vi "State Machine Automation.vi"() -> ()   [LabVIEW 2016]
panel:
  in  "Path":path=path "C:/Users/monke/OneDrive/Documents/Research/Repository/automation/itx folders/Destination Files"
  in  "Tab Control":enum32{"Conductance", "Transconductance"}(tab)
  out "Conductance":T1(graph)
  out "Cond. Intens. 2":dbl[][](graph)
  out "Transconductance":T1(graph)
  out "Trans. Intens. 2":dbl[][](graph)
  in  "STOP":bool
  out "Added?":string
  in  "Numeric":dbl=20.0
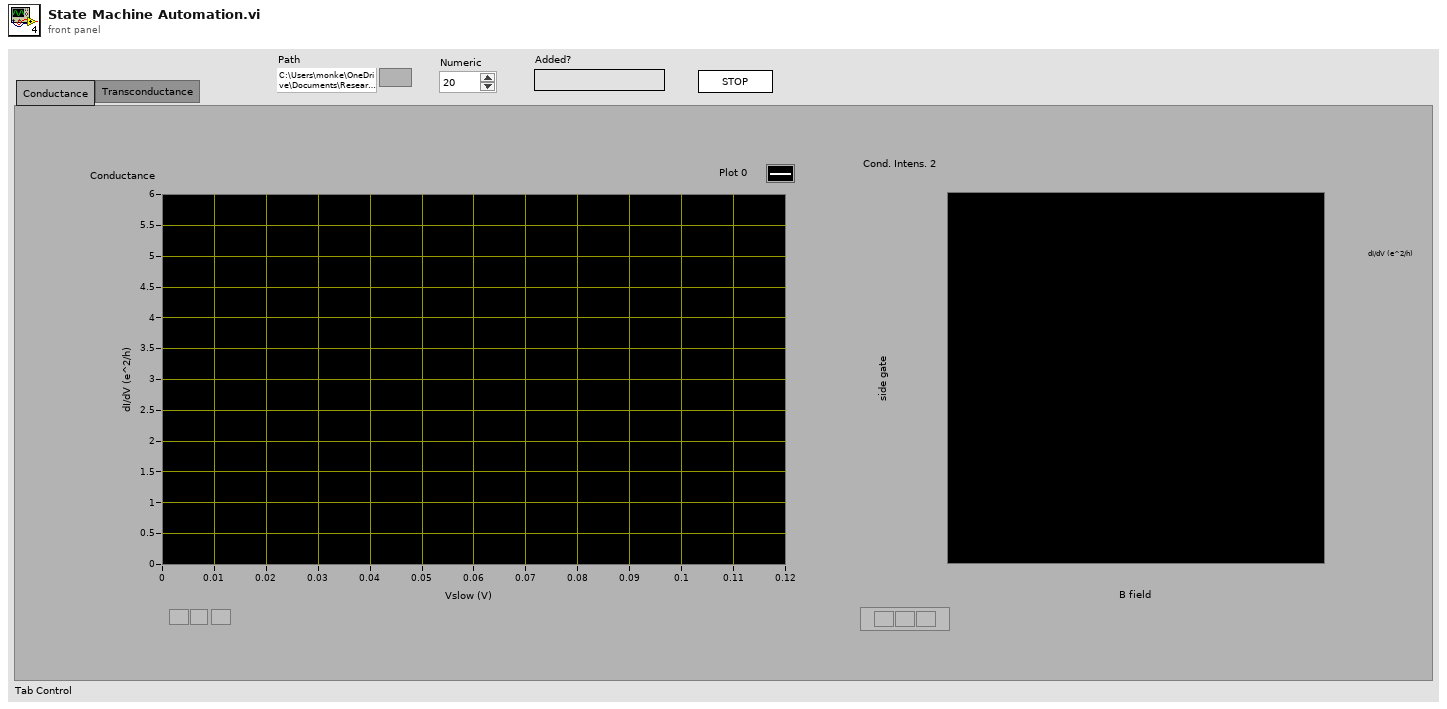
[diagram p1: front panel]
types:
  T1 = cluster{"Vfast":dbl[], "Decimated Array":dbl[]}[]
  T2 = enum32{"invalid app kind", "Development System", "Run Time System", "Student Edition", "Embedded LabVIEW", "Evaluation", "Custom"}
  T3 = enum32{"Invalid", "Standard", "Closed", "Hidden", "Minimized", "Maximized"}
  T4 = cluster{"Core":cluster{"Current VI Reference":refnum<vi>, "Close Panel on Exit?":bool}, "Your Boolean data":bool, "Your string data":string, "Path":path, "Normal Graphs":cluster{"A vs D":cluster{dbl[], dbl[]}[], "Transconductance 2":cluster{"Vfast":dbl[], "Decimated Array":dbl[]}[], "Start Up":cluster{dbl[], dbl[]}[]}, "Intensity Graphs":cluster{"Cond. Intens. 3":dbl[][], "Trans. Intens. 3":dbl[][]}, "offset":i32}
  T5 = cluster{"Cond. Intens. 3":dbl[][], "Trans. Intens. 3":dbl[][]}
  T6 = cluster{"A vs D":cluster{dbl[], dbl[]}[], "Transconductance 2":cluster{"Vfast":dbl[], "Decimated Array":dbl[]}[], "Start Up":cluster{dbl[], dbl[]}[]}
  T7 = cluster{"Current VI Reference":refnum<vi>, "Close Panel on Exit?":bool}
  T8 = cluster{"Decimated Array":dbl[], "Decimated Array":dbl[]}
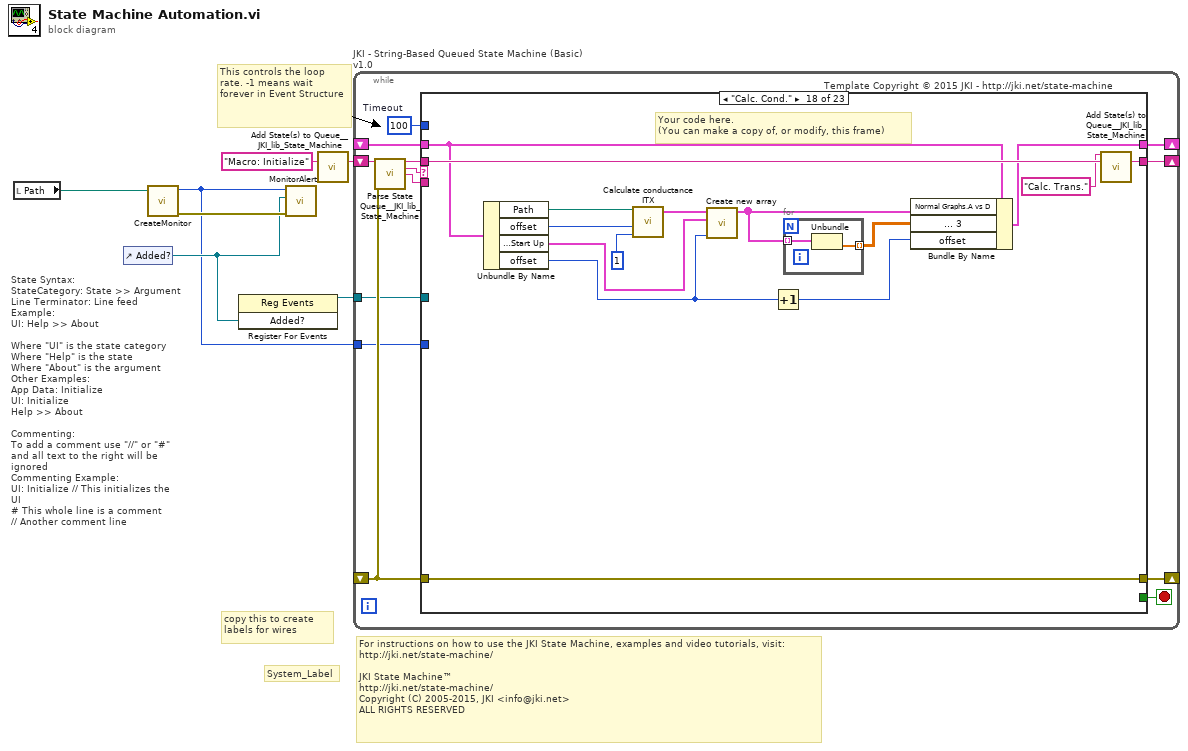
[diagram p0: block diagram]
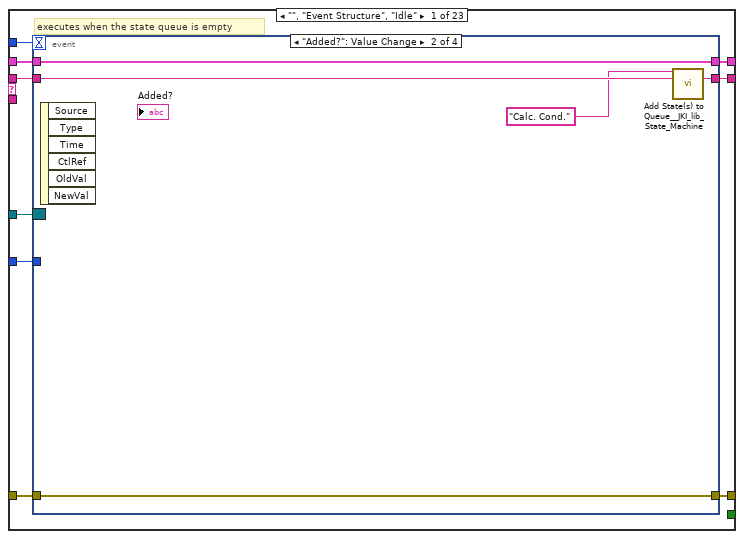
[diagram p2: hidden frame]
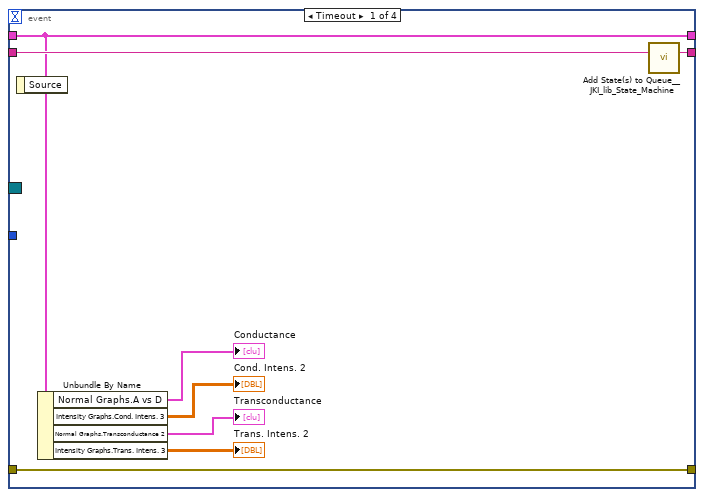
[diagram p3: hidden frame]
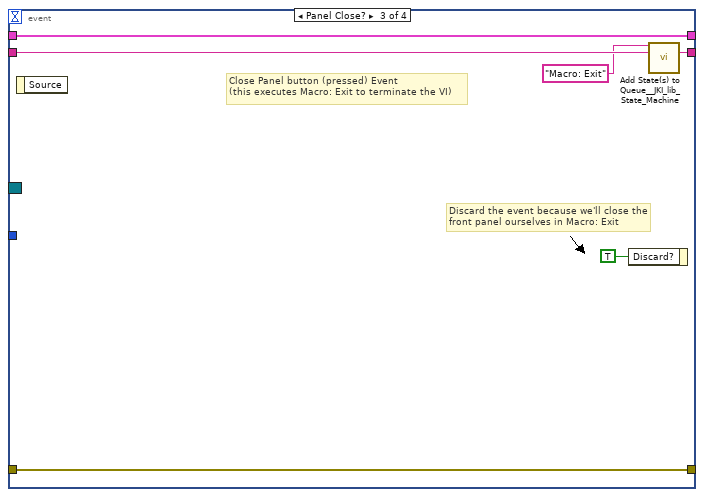
[diagram p4: hidden frame]
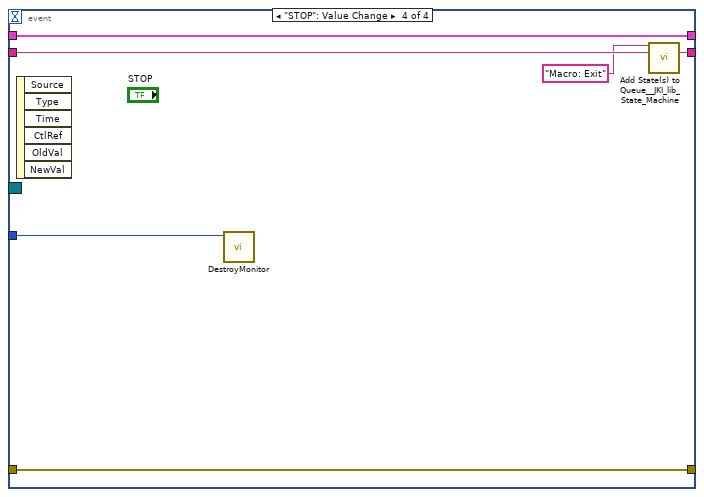
[diagram p5: hidden frame]
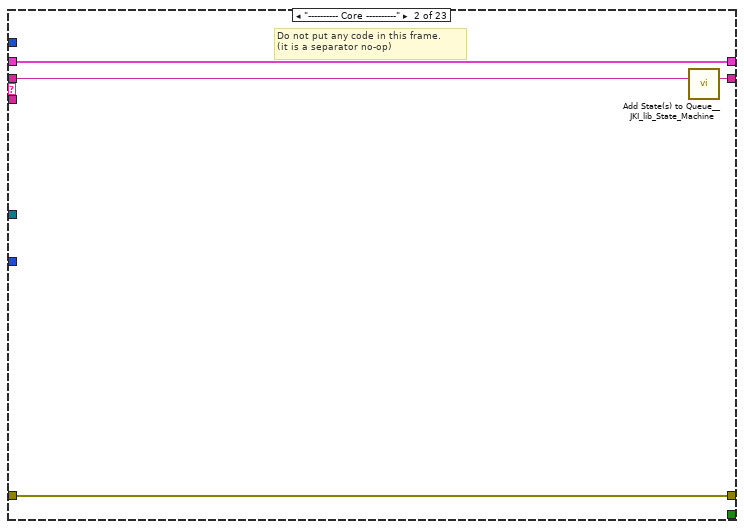
[diagram p6: hidden frame]
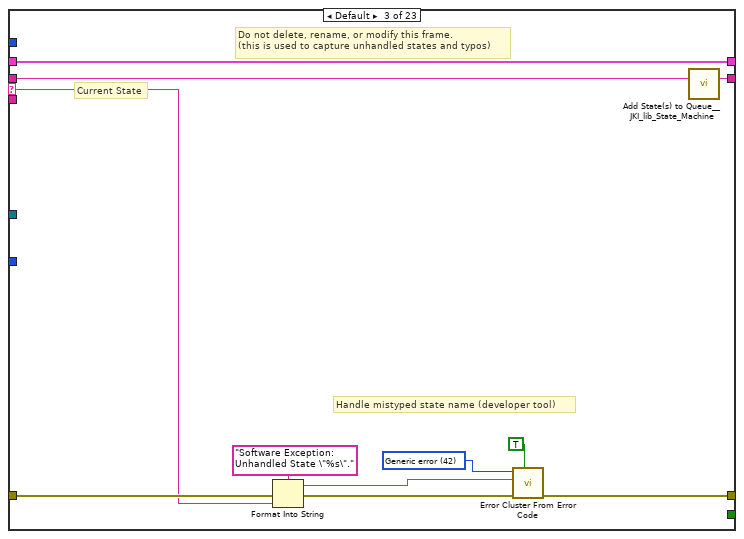
[diagram p7: hidden frame]
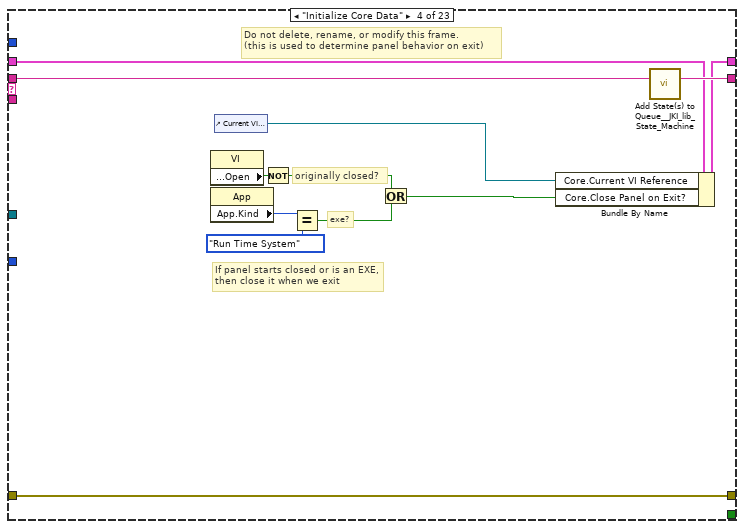
[diagram p8: hidden frame]
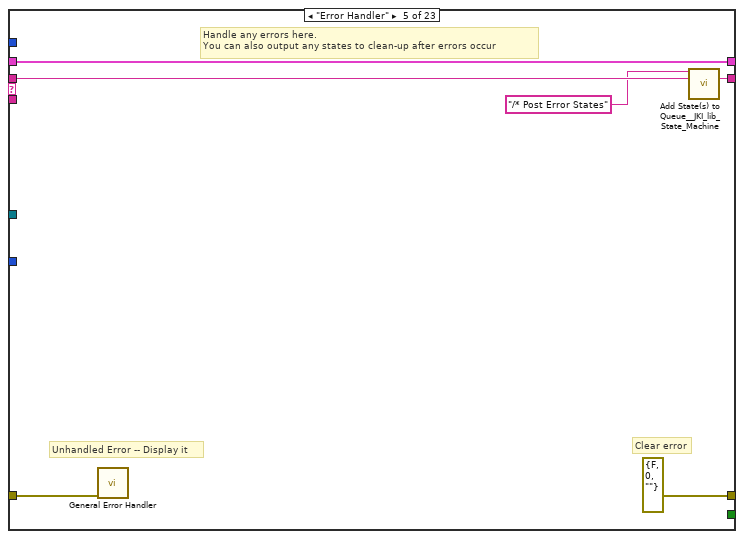
[diagram p9: hidden frame]
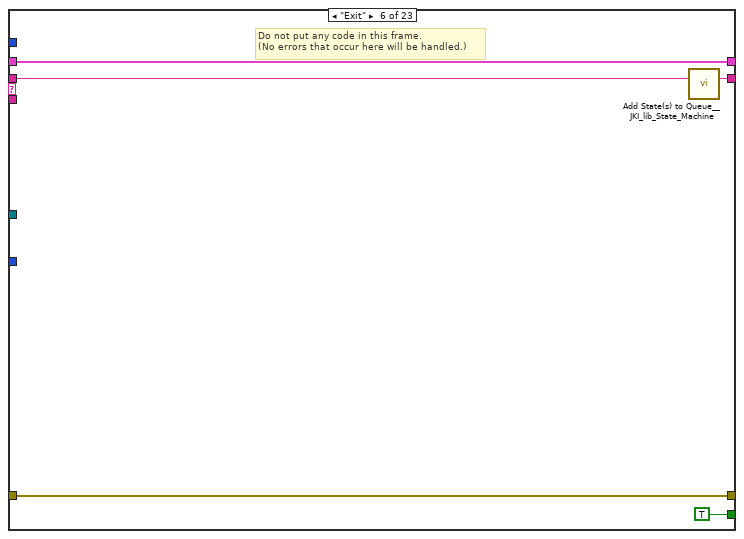
[diagram p10: hidden frame]
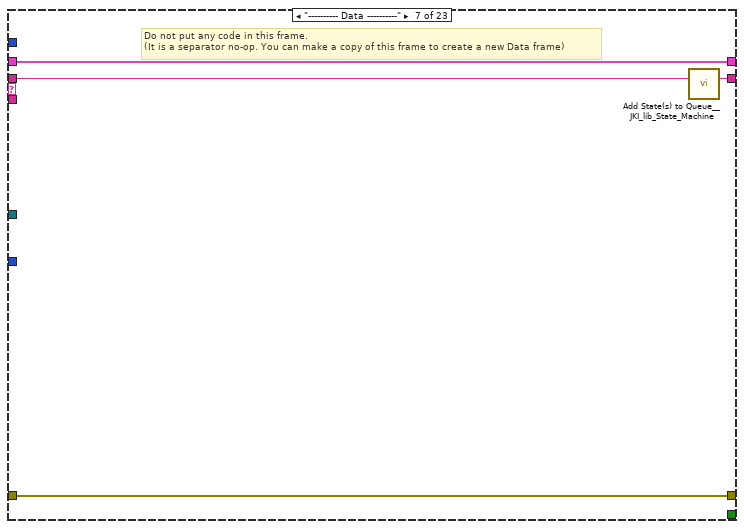
[diagram p11: hidden frame]
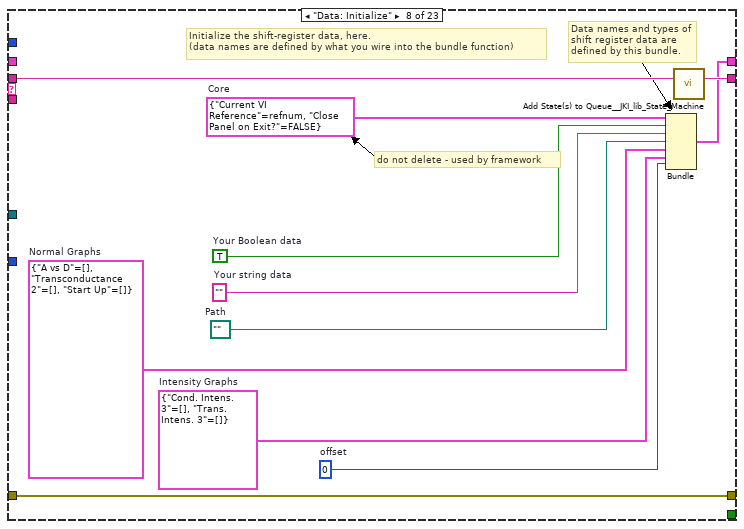
[diagram p12: hidden frame]
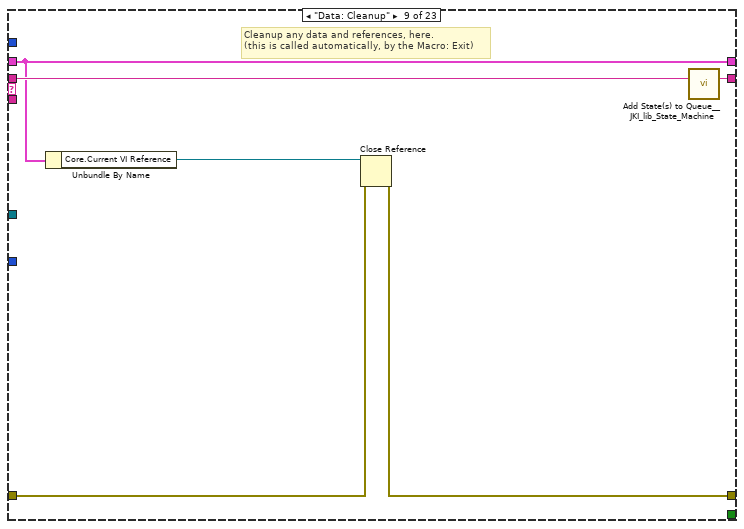
[diagram p13: hidden frame]
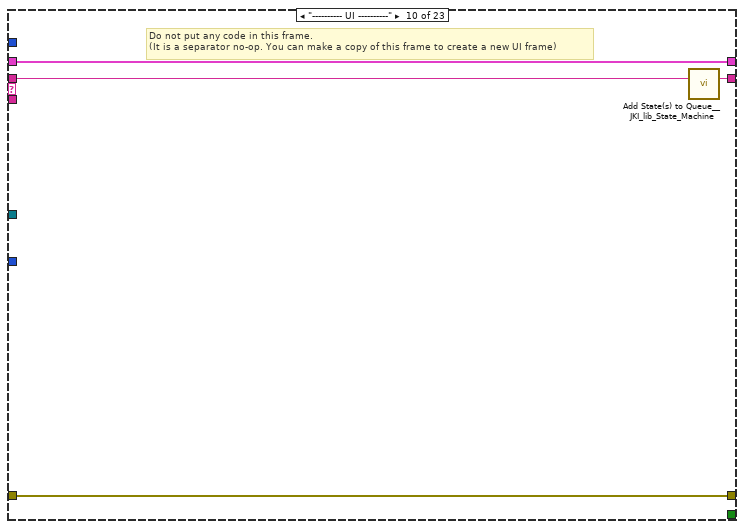
[diagram p14: hidden frame]
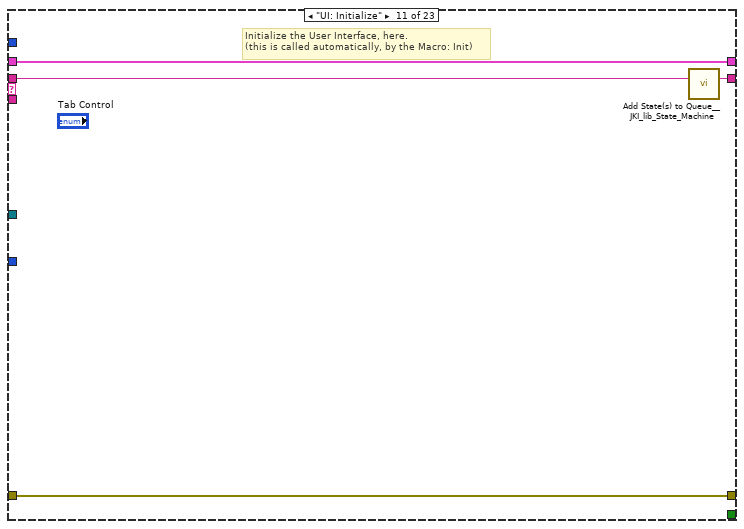
[diagram p15: hidden frame]
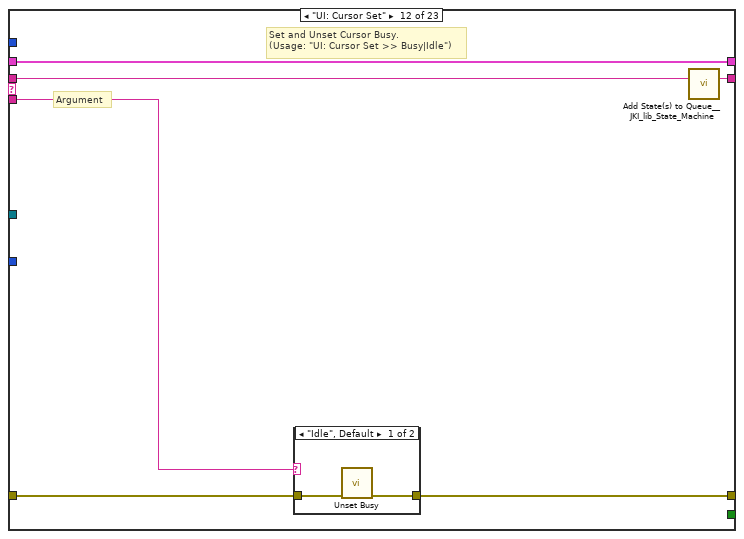
[diagram p16: hidden frame]
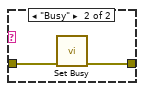
[diagram p17: hidden frame]
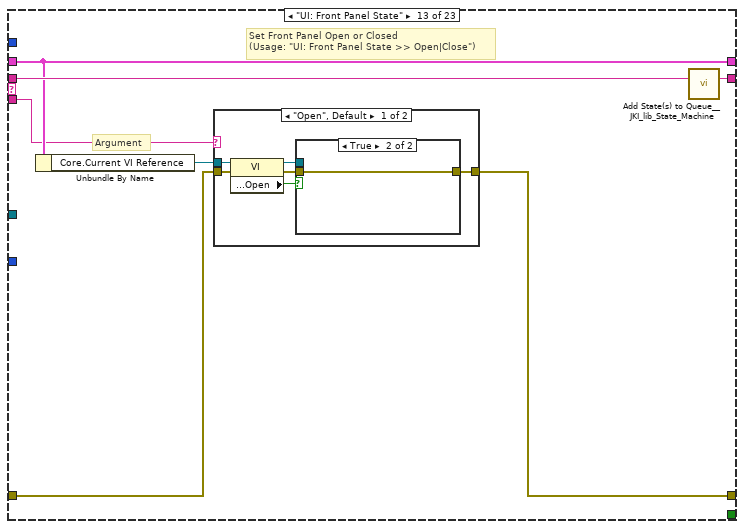
[diagram p18: hidden frame]
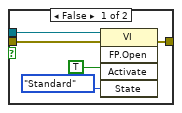
[diagram p19: hidden frame]
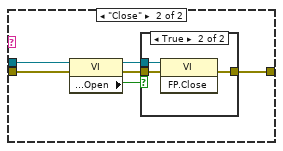
[diagram p20: hidden frame]
diagram:
  # "For instructions on how to use the JKI State Machine, examples and video tutorials, visit:\nhttp://jki.net/state-machine/\n\nJKI State Machine™\nhttp://jki.net/state-machine/\nCopyright (C) 2005-2015, JKI <info@jki.net>\nALL RIGHTS RESERVED"
  # "State Syntax:\nStateCategory: State >> Argument\nLine Terminator: Line feed\nExample:\nUI: Help >> About\n\nWhere \"UI\" is the state category\nWhere \"Help\" is the state\nWhere \"About\" is the argument\nOther Examples:\nApp Data: Initialize\nUI: Initialize\nHelp >> About\n\nCommenting:\nTo add a comment use \"//\" or \"#\" and all text to the right will be ignored\nCommenting Example:\nUI: Initialize // This initializes the UI\n# This whole line is a comment\n// Another comment line"
  # "copy this to create labels for wires"
  # "This controls the loop rate. -1 means wait forever in Event Structure"
  # "System_Label"
  n1 = local read "Path"() -> (w1:path)
  n2 = control-ref of="Added?"() -> (w4:refnum<vi>)
  n3 = call "CreateMonitor.vi"("File Path Control"=w1) -> ("error out"=w5:errorcluster, "Handle"=w2:i32)  [unwired: 9 in]
  n4 = register-events(w4) -> (reference out=w3:refnum<event-registration>)  [unwired: 2 in, 1 out]
  n5 = call "MonitorAlert.vi"("error in (no error)"=w5, "Str Refnum"=w4, "Handle"=w2) -> ()  [unwired: 8 in, 1 out]
  n6 = call <vilib>:"Add State(s) to Queue__JKI_lib_State_Machine.vi"("State(s) in (\"\")"="Macro: Initialize") -> ("States Out"=w7:string)  [unwired: 14 in]
  n7 = while "JKI - String-Based Queued State Machine (Basic) v1.0" {
    shift-right: [w13] -> _
    shift-left: _ -> [w12]
    shift-right: [w16] -> _
    shift-left: _ -> [w10]
    shift-right: [w15] -> _
    shift-left: w7 -> [w17]
    tunnel: w3 -> [w9]
    tunnel: w2 -> [w8]
    stop <- w14 stop-if-true
    w11 = 100  # Timeout
    # "Template Copyright © 2015 JKI - http://jki.net/state-machine"
    n8 = call <vilib>:"Parse State Queue__JKI_lib_State_Machine.vi"("State Queue"=w17, "Error In (no error)"=w10) -> ("Remaining States"=w19:string, "Current State"=w20:string, "Arguments"=w18:string)  [unwired: 11 in]
    n9 = case shown="\"Calc. Cond.\"" w20 {
      selector: w20 -> [_ _ w59 _ _ _ _ _ _ _ _ _ _ _ _ _ _ _ _ _ _ _ _]
      tunnel: w19 -> [w29 w58 w63 w81 w87 w92 w96 w107 w113 w117 w121 w127 w138 w164 w169 w179 w183 w198 w208 w217 w227 w231 w235]
      tunnel: w18 -> [_ _ _ _ _ _ _ _ _ _ _ w122 w132 _ _ _ _ _ _ _ _ _ _]
      tunnel: w12 -> [w27 w55 w61 w72 w84 w90 w93 _ w108 w114 w119 w125 w134 w161 w166 w176 w180 w194 w202 w214 w219 w228 w232]
      tunnel: [w26 w56 w65 w78 errorcluster {"status"=FALSE, "code"=0, "source"=""} ("error out") w89 w94 w104 w109 w115 w118 w123 w135 w162 w167 w177 w181 w196 w206 w215 w225 w229 w233] -> w16
      tunnel: w10 -> [w25 w56 w64 w78 w83 w89 w94 w104 w110 w115 w118 w124 w136 w162 w167 w177 w181 w196 w206 w215 w225 w229 w233]
      tunnel: [w28 w57 w62 w80 w86 w91 w95 w106 w112 w116 w120 w126 w137 w163 w168 w178 w182 w197 w207 w216 w226 w230 w234] -> w15
      tunnel: [_ _ _ _ _ TRUE _ _ _ _ _ _ _ _ _ _ _ _ _ _ _ _ _] -> w14
      tunnel: [w24 w55 w61 w79 w84 w90 w93 w105 w108 w114 w119 w125 w134 w161 w166 w176 w180 w193 w201 w214 w224 w228 w232] -> w13
      tunnel: w11 -> [w23 _ _ _ _ _ _ _ _ _ _ _ _ _ _ _ _ _ _ _ _ _ _]
      tunnel: w9 -> [w22 _ _ _ _ _ _ _ _ _ _ _ _ _ _ _ _ _ _ _ _ _ _]
      tunnel: w8 -> [w21 _ _ _ _ _ _ _ _ _ _ _ _ _ _ _ _ _ _ _ _ _ _]
      frame "", "Event Structure", "Idle" {
        # "executes when the state queue is empty"
        n10 = event shown="[1] \"Added?\": Value Change" {
          selector: w22 -> [_ _ _ _]
          dyn-events: _ -> [_ _ _ _]
          timeout: w23 -> [_ _ _ _]
          tunnel: w29 -> [w37 w42 w48 w54]
          tunnel: [w36 w41 w47 w53] -> w28
          tunnel: w27 -> [w30 w39 w45 w51]
          tunnel: [w35 w40 w46 w52] -> w26
          tunnel: w25 -> [w35 w40 w46 w52]
          tunnel: [w30 w39 w45 w51] -> w24
          tunnel: w21 -> [_ _ _ w49]
          event Timeout {
            n11 = event-data() -> ()  [unwired: 1 in, 1 out]
            n12 = Unbundle By Name(w30) -> ("Normal Graphs.A vs D"=→"Conductance":cluster{dbl[], dbl[]}[], "Intensity Graphs.Cond. Intens. 3"=→"Cond. Intens. 2":dbl[][], "Normal Graphs.Transconductance 2"=→"Transconductance":T1, "Intensity Graphs.Trans. Intens. 3"=→"Trans. Intens. 2":dbl[][])
            n13 = call <vilib>:"Add State(s) to Queue__JKI_lib_State_Machine.vi"("State(s) in (\"\")"=w37) -> ("States Out"=w36:string)  [unwired: 14 in]
          }
          event "Added?": Value Change {
            n14 = event-data() -> ()  [unwired: 1 in, 6 out]
            n15 = call <vilib>:"Add State(s) to Queue__JKI_lib_State_Machine.vi"("State(s) in Front (\"\")"="Calc. Cond." ("State(s) in Front (\"\")"), "State(s) in (\"\")"=w42) -> ("States Out"=w41:string)  [unwired: 13 in]
          }
          event Panel Close? {
            # "Discard the event because we'll close the front panel ourselves in Macro: Exit"
            # "Close Panel button (pressed) Event\n(this executes Macro: Exit to terminate the VI)"
            n16 = event-data() -> ()  [unwired: 1 in, 1 out]
            n17 = event-data("Discard?"=TRUE) -> ()  [unwired: 1 in, 1 out]
            n18 = call <vilib>:"Add State(s) to Queue__JKI_lib_State_Machine.vi"("State(s) in Front (\"\")"="Macro: Exit", "State(s) in (\"\")"=w48) -> ("States Out"=w47:string)  [unwired: 13 in]
          }
          event "STOP": Value Change {
            n19 = event-data() -> ()  [unwired: 1 in, 6 out]
            n20 = call "DestroyMonitor.vi"("Handle in"=w49) -> ()  [unwired: 10 in, 1 out]
            n21 = call <vilib>:"Add State(s) to Queue__JKI_lib_State_Machine.vi"("State(s) in Front (\"\")"="Macro: Exit", "State(s) in (\"\")"=w54) -> ("States Out"=w53:string)  [unwired: 13 in]
          }
        }
      }
      frame "---------- Core ----------" {
        # "Do not put any code in this frame.\n(it is a separator no-op)"
        n22 = call <vilib>:"Add State(s) to Queue__JKI_lib_State_Machine.vi"("State(s) in (\"\")"=w58) -> ("States Out"=w57:string)  [unwired: 14 in]
      }
      frame Default {
        w68 = 42 items=["No error", "Argument error", "Memory is full", "Out of zone", "End of file", "File already open", "Generic file I/O error", "File not found", "File permission error", "Disk is full", "Duplicate path", "Too many files open", "System feature not enabled", "Resource file not found", "Cannot add resource", "Resource not found", "Image not found", "Image memory error", "Pen does not exist", "Config type invalid", "Config token not found", "Config parse error", "Config memory error", "Bad external code format", "Bad external code offset", "External code not present", "Null window", "Destroy window error", "Null menu", "Print aborted", "Bad print record", "Print driver error", "Windows error during printing", "Memory error during printing", "Print dialog error", "Generic print error", "Invalid device refnum", "Device not found", "Device parameter error", "Device unit error", "Cannot open device", "Device call aborted", "Generic error", "Cancelled by user", "Object ID too low", "Object ID too high", "Object not in heap", "Unknown heap", "Unknown object (invalid DefProc)", "Unknown object (DefProc not in table)", "Message out of range", "Invalid (null) method", "Unknown message", "Manager call not supported", "Bad address", "Network operation in progress", "Network operation timed out", "Connection is busy", "Network attribute not supported", "Network error", "Address in use", "System out of memory", "Connection aborted", "Connection refused", "Not connected", "Already connected", "Connection closed", "Initialization error (interapplication manager)", "Bad occurrence", "Wait on unbound occurrence handler", "Occurrence queue overflow", "Datalog type conflict", "Unused", "Unrecognized type (interapplication manager)", "Memory corrupt", "Failed to make temporary DLL", "Old CIN version", "Drag socket not found", "Failed to load drop-object", "Failed to register OLE object", "Failed to release OLE object", "Format specifier type mismatch", "Unknown format specifier", "Too few format specifiers", "Too many format specifiers", "Scan failed", "Newer CIN version", "Error converting to variant", "Runtime menu error", "Password tampered", "Variant attribute not found", "Incompatible variant data type", "Event data is not available", "Event Store is not present", "Occurrence is not found", "Event Queue is not created", "Event info is not available", "Refnum passed is NULL", "Error retrieving Class GUID", "Error retrieving CoClass GUID", "Error retrieving TypeLib GUID.", "Bad built application magic bytes.", "Specific driver is different from the specific driver associated with the Logical Name.", "There is no session opened to the class driver.", "Max Error", "MAX - Error with config objects", "MAX - Error loading configuration", "MAX - Group not supported"]
        # "Current State"
        # "Do not delete, rename, or modify this frame.\n(this is used to capture unhandled states and typos)"
        # "Handle mistyped state name (developer tool)"
        n23 = Format Into String(format string="Software Exception: Unhandled State \"%s\"." ("message"), error in=w64, w59) -> (resulting string=w67:string, error out=w66:errorcluster)  [unwired: 1 in]
        n24 = call <vilib>:"Error Cluster From Error Code.vi"("show call chain? (False)"=TRUE, "error in (no error)"=w66, "error message (\"\")"=w67, "error code (0)"=w68) -> ("error out"=w65:errorcluster)  [unwired: 5 in]
        n25 = call <vilib>:"Add State(s) to Queue__JKI_lib_State_Machine.vi"("State(s) in (\"\")"=w63) -> ("States Out"=w62:string)  [unwired: 14 in]
      }
      frame "Initialize Core Data" {
        # "Do not delete, rename, or modify this frame.\n(this is used to determine panel behavior on exit)"
        # "originally closed?"
        # "exe?"
        # "If panel starts closed or is an EXE, then close it when we exit"
        n26 = property class="VI"() -> ("Front Panel.Open"=w77:bool)  [unwired: 2 in, 2 out]
        n27 = property class="App"() -> ("App.Kind"=w76:T2)  [unwired: 2 in, 2 out]
        n28 = control-ref of="Current VI Reference"() -> (w70:refnum<vi>)
        n29 = Not(x=w77) -> (.not. x?=w74:bool)
        n30 = Equal?(x=w76, y=T2."Run Time System" ("Application:Kind")) -> (x = y?=w73:bool)
        n31 = Or(x=w74, y=w73) -> (x .or. y?=w71:bool)
        n32 = Bundle By Name(cluster=w72, "Core.Current VI Reference"=w70, "Core.Close Panel on Exit?"=w71) -> (w79:T4)
        n33 = call <vilib>:"Add State(s) to Queue__JKI_lib_State_Machine.vi"("State(s) in (\"\")"=w81) -> ("States Out"=w80:string)  [unwired: 14 in]
      }
      frame "Error Handler" {
        # "Unhandled Error -- Display it"
        # "Handle any errors here.\nYou can also output any states to clean-up after errors occur"
        # "Clear error"
        n34 = call <vilib>:"General Error Handler.vi"("error in (no error)"=w83) -> ()  [unwired: 10 in, 5 out]
        n35 = call <vilib>:"Add State(s) to Queue__JKI_lib_State_Machine.vi"("State(s) in Front (\"\")"="/* Post Error States", "State(s) in (\"\")"=w87) -> ("States Out"=w86:string)  [unwired: 13 in]
      }
      frame "Exit" {
        # "Do not put any code in this frame.\n(No errors that occur here will be handled.)"
        n36 = call <vilib>:"Add State(s) to Queue__JKI_lib_State_Machine.vi"("State(s) in (\"\")"=w92) -> ("States Out"=w91:string)  [unwired: 14 in]
      }
      frame "---------- Data ----------" {
        # "Do not put any code in this frame.\n(It is a separator no-op. You can make a copy of this frame to create a new Data frame)"
        n37 = call <vilib>:"Add State(s) to Queue__JKI_lib_State_Machine.vi"("State(s) in (\"\")"=w96) -> ("States Out"=w95:string)  [unwired: 14 in]
      }
      frame "Data: Initialize" {
        w97 = 0  # offset
        w98 = T5 {"Cond. Intens. 3"=[], "Trans. Intens. 3"=[]}  # Intensity Graphs
        w99 = T6 {"A vs D"=[], "Transconductance 2"=[], "Start Up"=[]}  # Normal Graphs
        w100 = path ""  # Path
        w101 = T7 {"Current VI Reference"=refnum, "Close Panel on Exit?"=FALSE}  # Core
        w103 = TRUE  # Your Boolean data
        w102 = ""  # Your string data
        # "do not delete - used by framework"
        # "Data names and types of shift register data are defined by this bundle."
        # "Initialize the shift-register data, here.\n(data names are defined by what you wire into the bundle function)"
        n38 = Bundle("Core"=w101, "Your Boolean data"=w103, "Your string data"=w102, "Path"=w100, "Normal Graphs"=w99, "Intensity Graphs"=w98, "offset"=w97) -> (w105:T4)  [unwired: 1 in]
        n39 = call <vilib>:"Add State(s) to Queue__JKI_lib_State_Machine.vi"("State(s) in (\"\")"=w107) -> ("States Out"=w106:string)  [unwired: 14 in]
      }
      frame "Data: Cleanup" {
        # "Cleanup any data and references, here.\n(this is called automatically, by the Macro: Exit)"
        n40 = Unbundle By Name(w108) -> ("Core.Current VI Reference"=w111:refnum<vi>)
        n41 = Close Reference(reference=w111, error in (no error)=w110) -> (error out=w109:errorcluster)
        n42 = call <vilib>:"Add State(s) to Queue__JKI_lib_State_Machine.vi"("State(s) in (\"\")"=w113) -> ("States Out"=w112:string)  [unwired: 14 in]
      }
      frame "---------- UI ----------" {
        # "Do not put any code in this frame.\n(It is a separator no-op. You can make a copy of this frame to create a new UI frame)"
        n43 = call <vilib>:"Add State(s) to Queue__JKI_lib_State_Machine.vi"("State(s) in (\"\")"=w117) -> ("States Out"=w116:string)  [unwired: 14 in]
      }
      frame "UI: Initialize" {
        # "Initialize the User Interface, here.\n(this is called automatically, by the Macro: Init)"
        n44 = call <vilib>:"Add State(s) to Queue__JKI_lib_State_Machine.vi"("State(s) in (\"\")"=w121) -> ("States Out"=w120:string)  [unwired: 14 in]
      }
      frame "UI: Cursor Set" {
        # "Argument"
        # "Set and Unset Cursor Busy.\n(Usage: \"UI: Cursor Set >> Busy|Idle\")"
        n45 = case shown="\"Idle\", Default" w122 {
          tunnel: w124 -> [w129 w131]
          tunnel: [w128 w130] -> w123
          frame "Idle", Default {
            n46 = call <vilib>:"Unset Busy.vi"("error in (no error)"=w129) -> ("error out"=w128:errorcluster)  [unwired: 10 in]
          }
          frame "Busy" {
            n47 = call <vilib>:"Set Busy.vi"("error in (no error)"=w131) -> ("error out"=w130:errorcluster)  [unwired: 9 in, 1 out]
          }
        }
        n48 = call <vilib>:"Add State(s) to Queue__JKI_lib_State_Machine.vi"("State(s) in (\"\")"=w127) -> ("States Out"=w126:string)  [unwired: 14 in]
      }
      frame "UI: Front Panel State" {
        # "Argument"
        # "Set Front Panel Open or Closed\n(Usage: \"UI: Front Panel State >> Open|Close\")"
        n49 = Unbundle By Name(w134) -> ("Core.Current VI Reference"=w133:refnum<vi>)
        n50 = case shown="\"Open\", Default" w132 {
          tunnel: w136 -> [w142 w155]
          tunnel: [w144 w156] -> w135
          tunnel: w133 -> [w143 w153]
          frame "Open", Default {
            n51 = property class="VI"(reference=w143, error in=w142) -> (reference out=w140:refnum<vi>, error out=w141:errorcluster, "Front Panel.Open"=w139:bool)
            n52 = case shown="True" w139 {
              tunnel: [w147 w150] -> w144
              tunnel: w141 -> [w146 w150]
              tunnel: w140 -> [w145 _]
              frame False {
                n53 = invoke class="VI" method="FP.Open"(reference=w145, error in=w146, "Activate"=TRUE, "State"=T3."Standard") -> (error out=w147:errorcluster)  [unwired: 1 in, 4 out]
              }
              frame True {
              }
            }
          }
          frame "Close" {
            n54 = property class="VI"(reference=w153, error in=w155) -> (reference out=w152:refnum<vi>, error out=w154:errorcluster, "Front Panel.Open"=w151:bool)
            n55 = case shown="True" w151 {
              tunnel: [w157 w160] -> w156
              tunnel: w154 -> [w157 w159]
              tunnel: w152 -> [_ w158]
              frame False {
              }
              frame True {
                n56 = invoke class="VI" method="FP.Close"(reference=w158, error in=w159) -> (error out=w160:errorcluster)  [unwired: 1 in, 2 out]
              }
            }
          }
        }
        n57 = call <vilib>:"Add State(s) to Queue__JKI_lib_State_Machine.vi"("State(s) in (\"\")"=w138) -> ("States Out"=w137:string)  [unwired: 14 in]
      }
      frame "---------- Macro ----------" {
        # "Do not put any code in this frame.\n(It is a separator no-op. You can make a copy of this frame to create a new Macro frame)"
        n58 = call <vilib>:"Add State(s) to Queue__JKI_lib_State_Machine.vi"("State(s) in (\"\")"=w164) -> ("States Out"=w163:string)  [unwired: 14 in]
      }
      frame "Macro: Initialize" {
        # "Initialization Macro\n(This is called once, when the VI starts)"
        n59 = call <vilib>:"Add State(s) to Queue__JKI_lib_State_Machine.vi"("State(s) in Front (\"\")"="Data: Initialize\nInitialize Core Data\nUI: Initialize\nUI: Front Panel State >> Open\nCond.StartUp", "State(s) in (\"\")"=w169) -> ("States Out"=w168:string)  [unwired: 13 in]
      }
      frame "Macro: Exit" {
        # "Exit Macro\n(This is called once, when the VI exits)"
        n60 = Unbundle By Name(w176) -> ("Core.Close Panel on Exit?"=w175:bool)
        n61 = Select(t="UI: Front Panel State >> Close", s=w175, f="") -> (s? t:f=w172:string)
        n62 = call <vilib>:"Add State(s) to Queue__JKI_lib_State_Machine.vi"("State(s) in (\"\")"=w172, "State(s) at Back (\"\")"="Data: Cleanup\nExit") -> ("States Out"=w170:string)  [unwired: 13 in]
        n63 = call <vilib>:"Add State(s) to Queue__JKI_lib_State_Machine.vi"("State(s) in Front (\"\")"=w170, "State(s) in (\"\")"=w179) -> ("States Out"=w178:string)  [unwired: 13 in]
      }
      frame "---------- Cond. Trans. ----------" {
        # "Template Separator\n(You can make a copy of, or modify, this frame)"
        n64 = call <vilib>:"Add State(s) to Queue__JKI_lib_State_Machine.vi"("State(s) in (\"\")"=w183) -> ("States Out"=w182:string)  [unwired: 14 in]
      }
      frame "Calc. Cond." {
        # "Your code here.\n(You can make a copy of, or modify, this frame)"
        n65 = Unbundle By Name(w194) -> ("Path"=w195:path, "offset"=w186:i32, "Normal Graphs.Start Up"=w187:cluster{dbl[], dbl[]}[], "offset"=w185:i32)
        n66 = call "Calculate conductance ITX.vi"("length"=1, "offset"=w186, "File or Folder Path"=w195) -> ("A vs D"=w189:cluster{dbl[], dbl[]}[])  [unwired: 1 in, 3 out]
        n67 = call "Create new array.vi"("Numeric"=w185, "Array 2"=w187, "A vs D"=w189) -> ("Array"=w184:cluster{dbl[], dbl[]}[])  [unwired: 8 in]
        n68 = Increment(x=w185) -> (x+1=w188:i32)
        n69 = for {
          tunnel: w184 -> [w200] mode=indexing
          tunnel: [w199] -> w191 mode=indexing
          n70 = Unbundle(w200) -> (w199:dbl[])  [unwired: 1 out]
        }
        n71 = Bundle By Name(cluster=w194, "Normal Graphs.A vs D"=w184, "Intensity Graphs.Cond. Intens. 3"=w191, "offset"=w188) -> (w193:T4)
        n72 = call <vilib>:"Add State(s) to Queue__JKI_lib_State_Machine.vi"("State(s) in Front (\"\")"="Calc. Trans." ("State(s) in Front (\"\")"), "State(s) in (\"\")"=w198) -> ("States Out"=w197:string)  [unwired: 13 in]
      }
      frame "Calc. Trans." {
        n73 = Unbundle By Name(w202) -> ("Normal Graphs.A vs D"=w205:cluster{dbl[], dbl[]}[])
        n74 = for {
          tunnel: w205 -> [w213] mode=indexing
          tunnel: [w210] -> w204 mode=indexing
          tunnel: [w209] -> w203 mode=indexing
          n75 = call <userlib>:"differential.vi"("Numeric"="Numeric", "dy/dx vs x"=TRUE, "A vs B 2"=w213) -> ("A vs B 3"=w210:T8)  [unwired: 1 in]
          n76 = Unbundle(w210) -> ("Decimated Array"=w209:dbl[])  [unwired: 1 out]
        }
        n77 = Bundle By Name(cluster=w202, "Normal Graphs.Transconductance 2"=w204, "Intensity Graphs.Trans. Intens. 3"=w203) -> (w201:T4)
        n78 = call <vilib>:"Add State(s) to Queue__JKI_lib_State_Machine.vi"("State(s) in (\"\")"=w208) -> ("States Out"=w207:string)  [unwired: 14 in]
      }
      frame "---------- Start Up ----------" {
        # "Template Separator\n(You can make a copy of, or modify, this frame)"
        n79 = call <vilib>:"Add State(s) to Queue__JKI_lib_State_Machine.vi"("State(s) in (\"\")"=w217) -> ("States Out"=w216:string)  [unwired: 14 in]
      }
      frame "Cond.StartUp" {
        n80 = call "Calculate conductance ITX.vi"("length"=1000, "offset"=0, "File or Folder Path"="Path") -> ("A vs D"=w220:cluster{dbl[], dbl[]}[])  [unwired: 1 in, 3 out]
        n81 = Array Size(array=w220) -> (size(s)=w223:i32)
        n82 = Bundle By Name(cluster=w219, "Path"="Path", "Normal Graphs.Start Up"=w220, "offset"=w223) -> (w224:T4)
        n83 = call <vilib>:"Add State(s) to Queue__JKI_lib_State_Machine.vi"("State(s) in (\"\")"=w227) -> ("States Out"=w226:string)  [unwired: 14 in]
      }
      frame "---------- Copy Me ----------" {
        # "Template Separator\n(You can make a copy of, or modify, this frame)"
        n84 = call <vilib>:"Add State(s) to Queue__JKI_lib_State_Machine.vi"("State(s) in (\"\")"=w231) -> ("States Out"=w230:string)  [unwired: 14 in]
      }
      frame "Copy Me" {
        # "Your code here.\n(You can make a copy of, or modify, this frame)"
        n85 = call <vilib>:"Add State(s) to Queue__JKI_lib_State_Machine.vi"("State(s) in (\"\")"=w235) -> ("States Out"=w234:string)  [unwired: 14 in]
      }
    }
  }
